vi "multiply.vi"(2 "INPUT_B":T2, 3 "INPUT_A":T2) -> (0 "OUTPUT":T1, 1 "OVERFLOW":bool)   [LabVIEW 2013]
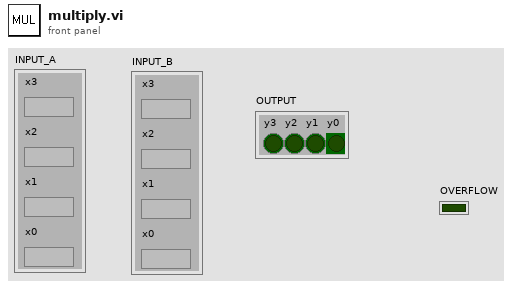
[diagram p1: front panel]
types:
  T1 = cluster{"y3":bool, "y2":bool, "y1":bool, "y0":bool}
  T2 = cluster{"x3":bool, "x2":bool, "x1":bool, "x0":bool}
  T3 = cluster{"x0":bool, "x1":bool, "x2":bool, "x3":bool}
  T4 = cluster{"X 0":bool, "X 1":bool, "X 2":bool, "X 3":bool}
  T5 = cluster{"X 1":bool, "X 2":bool, "X 3":bool, bool}
  T6 = cluster{"q0":bool, "q0":bool, "q0":bool, "X 0":bool}
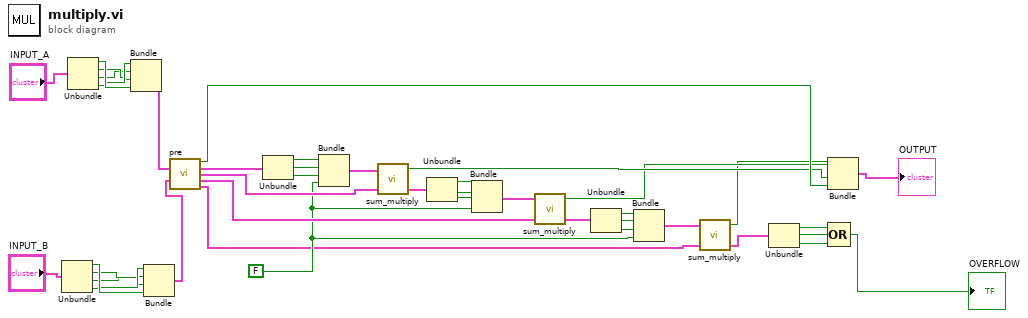
[diagram p0: block diagram]
diagram:
  w9 = FALSE
  n1 = Unbundle("INPUT_B") -> ("x3"=w25:bool, "x2"=w23:bool, "x1"=w22:bool, "x0"=w24:bool)
  n2 = Unbundle("INPUT_A") -> ("x3"=w29:bool, "x2"=w27:bool, "x1"=w26:bool, "x0"=w28:bool)
  n3 = Bundle("x0"=w28, "x1"=w26, "x2"=w27, "x3"=w29) -> (w33:T3)  [unwired: 1 in]
  n4 = Bundle("x0"=w24, "x1"=w22, "x2"=w23, "x3"=w25) -> (w32:T3)  [unwired: 1 in]
  n5 = call "pre.vi"("A"=w33, "B"=w32) -> ("X 0"=w4:bool, "P 1"=w41:cluster{"X 1":bool, "X 2":bool, "X 3":bool}, "P 2"=w20:T4, "P 3"=w14:T4, "P 4"=w7:T4)  [unwired: 9 in]
  n6 = Unbundle(w41) -> ("X 1"=w40:bool, "X 2"=w39:bool, "X 3"=w38:bool)
  n7 = Bundle("X 1"=w40, "X 2"=w39, "X 3"=w38, w9) -> (w21:T5)  [unwired: 1 in]
  n8 = call "sum_multiply.vi"("Pi"=w20, "Pi-1"=w21) -> ("S"=w19:cluster{"s0":bool, "s1":bool, "s2":bool}, "q0"=w3:bool)  [unwired: 2 in]
  n9 = Unbundle(w19) -> ("s0"=w18:bool, "s1"=w17:bool, "s2"=w16:bool)
  n10 = Bundle("s0"=w18, "s1"=w17, "s2"=w16, w9) -> (w15:cluster{"s0":bool, "s1":bool, "s2":bool, bool})  [unwired: 1 in]
  n11 = call "sum_multiply.vi"("Pi"=w14, "Pi-1"=w15) -> ("S"=w13:cluster{"s0":bool, "s1":bool, "s2":bool}, "q0"=w2:bool)  [unwired: 2 in]
  n12 = Unbundle(w13) -> ("s0"=w12:bool, "s1"=w11:bool, "s2"=w10:bool)
  n13 = Bundle("s0"=w12, "s1"=w11, "s2"=w10, w9) -> (w8:cluster{"s0":bool, "s1":bool, "s2":bool, bool})  [unwired: 1 in]
  n14 = call "sum_multiply.vi"("Pi"=w7, "Pi-1"=w8) -> ("S"=w6:cluster{"s0":bool, "s1":bool, "s2":bool}, "q0"=w1:bool)  [unwired: 2 in]
  n15 = Unbundle(w6) -> ("s0"=w37:bool, "s1"=w36:bool, "s2"=w35:bool)
  n16 = Bundle("q0"=w1, "q0"=w2, "q0"=w3, "X 0"=w4) -> (→"OUTPUT":T6)  [unwired: 1 in]
  n17 = Compound Arithmetic op=OR(w37, w36, w35) -> (→"OVERFLOW":bool)
